vi "Close Video Capture.vi"() -> (0 "error code OUT":i32)   [LabVIEW 2013]
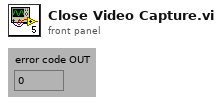
[diagram p1: front panel]
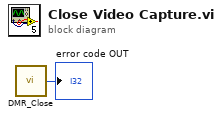
[diagram p0: block diagram]
diagram:
  n1 = call "DMR_Close.vi"() -> ("error code OUT"=→"error code OUT":i32)
